vi "xcamera-make_trigger-mode-frame-start.vi"(11 "Option":enum16{"Off", "On"}(ring)) -> (3 "Serial String":string)   [LabVIEW 2012]
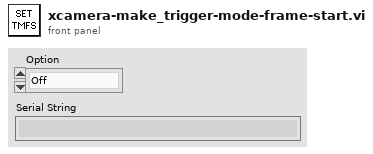
[diagram p1: front panel]
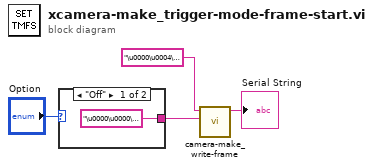
[diagram p0: block diagram]
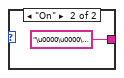
[diagram p2: hidden frame]
diagram:
  n1 = case shown="\"Off\"" "Option" {
    tunnel: ["\u0000\u0000\u0000\u0000" ("Address") "\u0000\u0000\u0000\u0001" ("Address")] -> w1
    frame "Off" {
    }
    frame "On" {
    }
  }
  n2 = call "camera-make_write-frame.vi"("Data"=w1, "Address"="\u0000\u0004\u0002\u0000") -> ("Serial String"=→"Serial String":string)  [unwired: 9 in]
